vi "和校验-8.vi"(8 "错误输入":errorcluster caption="错误输入（无错误）", 11 "需校验字符串":string) -> (0 "错误输出":errorcluster, 3 "校验":string)   [LabVIEW 2013, in "校验.lvlib"]
doc: "<B>输入端子 需校验字符串 ：</B>输入需要校验的字符串\n<B>输出端子 校验：</B>将需要校验的字符串，通过校验和-8算法，求出校验\n\n公式：将字符串两两拆分，然后相加，最后除以256.\n编写人：曾嘉康\n编写时间：2014/12/18"
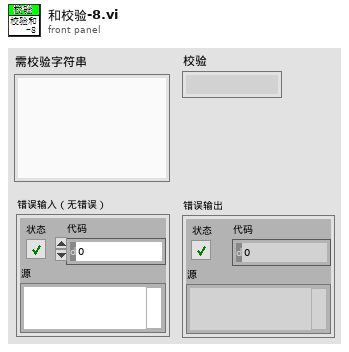
[diagram p1: front panel]
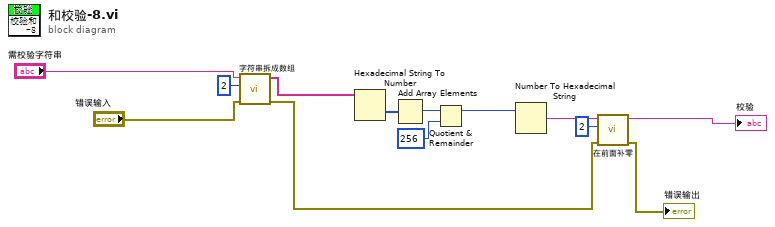
[diagram p0: block diagram]
diagram:
  n1 = call "字符串拆成数组.vi"("错误输入"="错误输入", "索引"=2, "字符串"="需校验字符串") -> ("错误输出"=w1:errorcluster, "数组"=w6:string[])  [unwired: 7 in]
  n2 = Hexadecimal String To Number(string=w6) -> (number=w11:u32[])  [unwired: 2 in, 1 out]
  n3 = Add Array Elements(numeric array=w11) -> (sum=w10:u32)
  n4 = Quotient & Remainder(x=w10, y=u32 256) -> (x-y*floor(x/y)=w7:u32)  [unwired: 1 out]
  n5 = Number To Hexadecimal String(2:w7) -> (0:w8:string)  [unwired: 1 in]
  n6 = call-poly "在前面补零.vi"("error in (no error)"=w1, "需达到的长度"=2, "字符串输入"=w8) -> ("error out"=→"错误输出":errorcluster, "连接的字符串"=→"校验":string)  [unwired: 7 in]
